vi "solar_voy Get Bits (COSMOS).vi"(6 "Bit Element Size (Array only)":i32, 7 "Endian (BIG)":enum8{"BIG", "LITTLE"}(ring), 8 "COSMOS TYPE":T1, 9 "Bit Size":i32, 10 "Bit Offset":i32, 11 "COSMOS Data":string) -> (2 "Bit Offset Past Value":i32, 3 "LabVIEW Flattened Value":string)   [LabVIEW 2018]
doc: "This unpacks the COSMOS Data given the bit offset and bit size into a LabVIEW Flattened Value."
uses:
  solar_voy_def/solar_voy_def_ctl ITEM TYPE.ctl
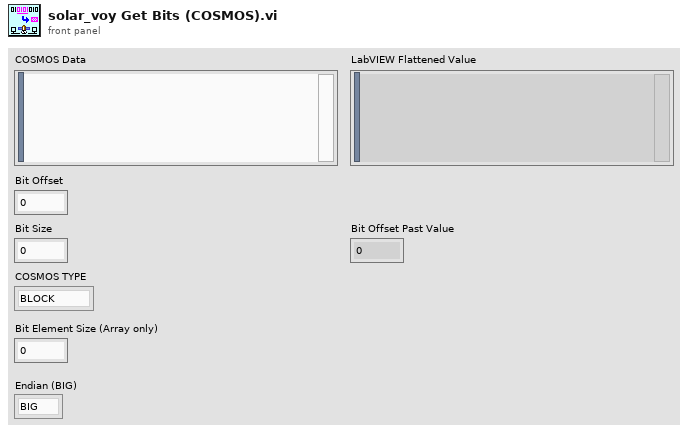
[diagram p1: front panel]
types:
  T1 = typedef "solar_voy_def_ctl ITEM TYPE.ctl" = enum8{"BLOCK", "INT", "UINT", "FLOAT", "STRING"}
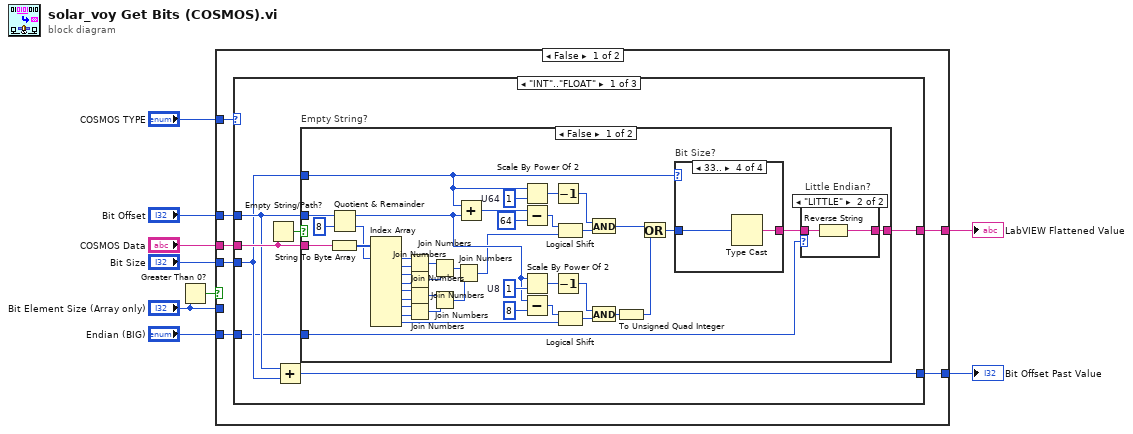
[diagram p0: block diagram]
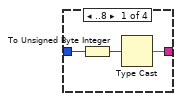
[diagram p3: hidden frame]
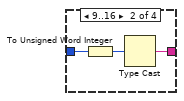
[diagram p4: hidden frame]
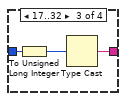
[diagram p5: hidden frame]
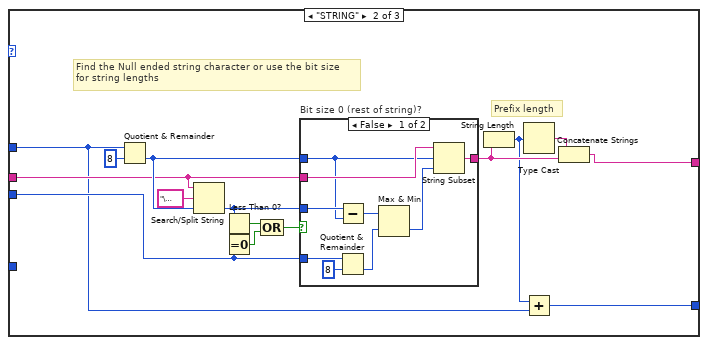
[diagram p7: hidden frame]
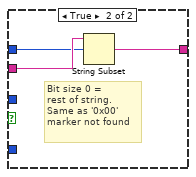
[diagram p8: hidden frame]
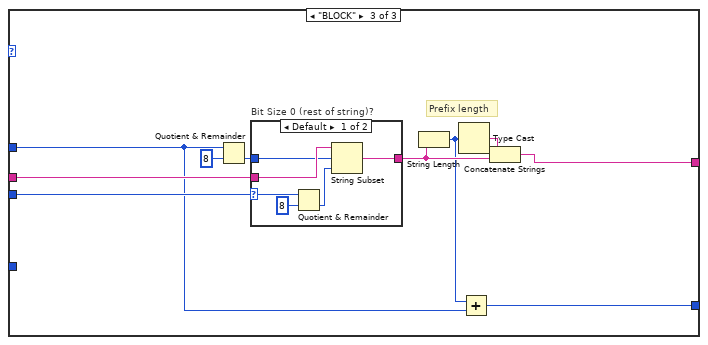
[diagram p9: hidden frame]
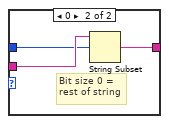
[diagram p10: hidden frame]
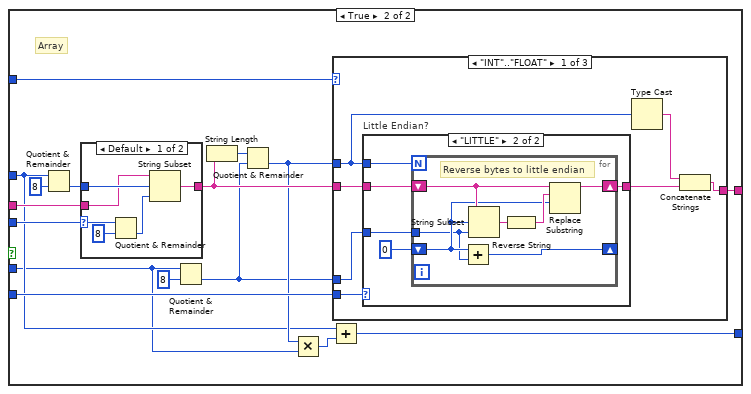
[diagram p11: hidden frame]
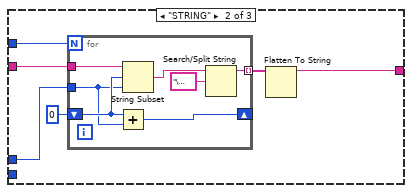
[diagram p13: hidden frame]
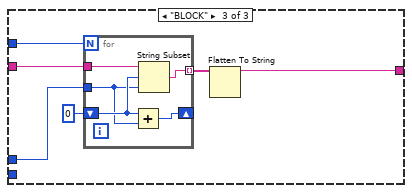
[diagram p14: hidden frame]
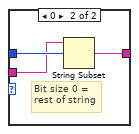
[diagram p15: hidden frame]
diagram:
  n1 = Greater Than 0?(x="Bit Element Size (Array only)") -> (x > 0?=w1:bool)
  n2 = case shown="False" w1 {
    tunnel: "COSMOS Data" -> [w16 w140]
    tunnel: [w15 w136] -> w8
    tunnel: "Bit Offset" -> [w14 w129]
    tunnel: "Bit Size" -> [w13 w139]
    tunnel: [w12 w128] -> w5
    tunnel: "COSMOS TYPE" -> [w11 w137]
    tunnel: "Endian (BIG)" -> [w10 w135]
    tunnel: "Bit Element Size (Array only)" -> [_ w127]
    frame False {
      n3 = case shown="\"INT\"..\"FLOAT\"" w11 {
        tunnel: w16 -> [w23 w88 w115]
        tunnel: [w22 w85 w111] -> w15
        tunnel: w14 -> [w21 w82 w109]
        tunnel: w13 -> [w20 w87 w112]
        tunnel: [w19 w81 w108] -> w12
        tunnel: w10 -> [w17 _ _]
        frame "INT".."FLOAT" {
          n4 = Empty String/Path?(string/path=w23) -> (empty?=w18:bool)
          n5 = Add(x=w21, y=w20) -> (x+y=w19:i32)
          n6 = case "Empty String?" shown="False" w18 {
            tunnel: w23 -> [w55 _]
            tunnel: [w25 _] -> w22
            tunnel: w21 -> [w65 _]
            tunnel: w20 -> [w64 _]
            tunnel: w17 -> [w24 _]
            frame False {
              w38 = u8 1  # U8
              w59 = u64 1  # U64
              n7 = String To Byte Array(string=w55) -> (unsigned byte array=w54:u8[])
              n8 = Quotient & Remainder(x=w65, y=8) -> (x-y*floor(x/y)=w37:i32, floor(x/y)=w27:i32)
              n9 = Index Array(array=w54, index #1=w27) -> (element #1=w53:u8, element #2=w52:u8, element #3=w51:u8, element #4=w50:u8, element #5=w49:u8, element #6=w48:u8, element #7=w47:u8, element #8=w46:u8, element #9=w33:u8)  [unwired: 8 in]
              n10 = Join Numbers(hi=w53, lo=w52) -> ((hi.lo)=w45:u16)
              n11 = Join Numbers(hi=w51, lo=w50) -> ((hi.lo)=w43:u16)
              n12 = Join Numbers(hi=w49, lo=w48) -> ((hi.lo)=w44:u16)
              n13 = Join Numbers(hi=w47, lo=w46) -> ((hi.lo)=w42:u16)
              n14 = Join Numbers(hi=w45, lo=w43) -> ((hi.lo)=w41:u32)
              n15 = Join Numbers(hi=w44, lo=w42) -> ((hi.lo)=w40:u32)
              n16 = Join Numbers(hi=w41, lo=w40) -> ((hi.lo)=w26:u64)
              n17 = Add(x=w64, y=w37) -> (x+y=w62:i32)
              n18 = Scale By Power Of 2(n=w64, x=w59) -> (x*2^n=w58:u64)
              n19 = Subtract(x=w62, y=64) -> (x-y=w56:i32)
              n20 = Scale By Power Of 2(n=w37, x=w38) -> (x*2^n=w39:u8)
              n21 = Subtract(x=w37, y=8) -> (x-y=w34:i32)
              n22 = Decrement(x=w58) -> (x-1=w57:u64)
              n23 = Decrement(x=w39) -> (x-1=w35:u8)
              n24 = Logical Shift(y=w56, x=w26) -> (x << y=w60:u64)
              n25 = Logical Shift(y=w34, x=w33) -> (x << y=w32:u8)
              n26 = And(x=w57, y=w60) -> (x .and. y?=w29:u64)
              n27 = And(x=w35, y=w32) -> (x .and. y?=w31:u8)
              n28 = To Unsigned Quad Integer(1:w31) -> (0:w30:u64)
              n29 = Or(x=w29, y=w30) -> (x .or. y?=w28:u64)
              n30 = case "Bit Size?" shown="33.." w64 {
                tunnel: [w72 w75 w78 w80] -> w66
                tunnel: w28 -> [w71 w74 w77 w79]
                frame ..8 {
                  n31 = To Unsigned Byte Integer(number=w71) -> (unsigned 8bit integer=w70:u8)
                  n32 = Type Cast(x=w70) -> (*(type *) &x=w72:string)  [unwired: 1 in]
                }
                frame 9..16 {
                  n33 = To Unsigned Word Integer(number=w74) -> (unsigned 16bit integer=w73:u16)
                  n34 = Type Cast(x=w73) -> (*(type *) &x=w75:string)  [unwired: 1 in]
                }
                frame 17..32 {
                  n35 = To Unsigned Long Integer(number=w77) -> (unsigned 32bit integer=w76:u32)
                  n36 = Type Cast(x=w76) -> (*(type *) &x=w78:string)  [unwired: 1 in]
                }
                frame 33.. {
                  n37 = Type Cast(x=w79) -> (*(type *) &x=w80:string)  [unwired: 1 in]
                }
              }
              n38 = case "Little Endian?" shown="\"LITTLE\"" w24 {
                tunnel: w66 -> [w67 w69]
                tunnel: [w67 w68] -> w25
                frame "BIG", Default {
                }
                frame "LITTLE" {
                  n39 = Reverse String(1:w69) -> (0:w68:string)
                }
              }
            }
            frame True {
            }
          }
        }
        frame "STRING" {
          # "Find the Null ended string character or use the bit size\nfor string lengths"
          # "Prefix length"
          n40 = Quotient & Remainder(x=w82, y=8) -> (floor(x/y)=w93:i32)  [unwired: 1 out]
          n41 = Search/Split String(string=w88, search string/char (-)="\u0000", offset (0)=w93) -> (offset of match=w92:i32)  [unwired: 2 out]
          n42 = Less Than 0?(x=w92) -> (x < 0?=w91:bool)
          n43 = Equal To 0?(x=w87) -> (x = 0?=w90:bool)
          n44 = Compound Arithmetic op=OR(w91, w90) -> (w89:bool)
          n45 = case "Bit size 0 (rest of string)?" shown="False" w89 {
            tunnel: w88 -> [w104 w107]
            tunnel: w92 -> [w103 _]
            tunnel: w93 -> [w102 w106]
            tunnel: [w97 w105] -> w84
            tunnel: w87 -> [w96 _]
            frame False {
              n46 = Subtract(x=w103, y=w102) -> (x-y=w100:i32)
              n47 = Quotient & Remainder(x=w96, y=8) -> (floor(x/y)=w99:i32)  [unwired: 1 out]
              n48 = Max & Min(x=w100, y=w99) -> (min(x,y)=w98:i32)  [unwired: 1 out]
              n49 = String Subset(string=w104, offset (0)=w102, length (rest)=w98) -> (substring=w97:string)
            }
            frame True {
              # "Bit size 0 =\nrest of string.\nSame as '0x00'\nmarker not found"
              n50 = String Subset(string=w107, offset (0)=w106) -> (substring=w105:string)  [unwired: 1 in]
            }
          }
          n51 = String Length(string=w84) -> (length=w83:i32)
          n52 = Type Cast(x=w83) -> (*(type *) &x=w86:string)  [unwired: 1 in]
          n53 = Add(x=w83, y=w82) -> (x+y=w81:i32)
          n54 = Concatenate Strings(w86, w84) -> (w85:string)
        }
        frame "BLOCK" {
          # "Prefix length"
          n55 = Quotient & Remainder(x=w109, y=8) -> (floor(x/y)=w116:i32)  [unwired: 1 out]
          n56 = case "Bit Size 0 (rest of string)?" shown="Default" w112 {
            selector: w112 -> [w118 _]
            tunnel: w115 -> [w123 w126]
            tunnel: w116 -> [w122 w124]
            tunnel: [w121 w125] -> w113
            frame Default {
              n57 = Quotient & Remainder(x=w118, y=8) -> (floor(x/y)=w120:i32)  [unwired: 1 out]
              n58 = String Subset(string=w123, offset (0)=w122, length (rest)=w120) -> (substring=w121:string)
            }
            frame 0 {
              # "Bit size 0 =\nrest of string"
              n59 = String Subset(string=w126, offset (0)=w124) -> (substring=w125:string)  [unwired: 1 in]
            }
          }
          n60 = String Length(string=w113) -> (length=w110:i32)
          n61 = Type Cast(x=w110) -> (*(type *) &x=w114:string)  [unwired: 1 in]
          n62 = Add(x=w110, y=w109) -> (x+y=w108:i32)
          n63 = Concatenate Strings(w114, w113) -> (w111:string)
        }
      }
    }
    frame True {
      # "Array"
      n64 = Quotient & Remainder(x=w129, y=8) -> (floor(x/y)=w142:i32)  [unwired: 1 out]
      n65 = case shown="Default" w139 {
        selector: w139 -> [w187 _]
        tunnel: w142 -> [w192 w195]
        tunnel: w140 -> [w190 w194]
        tunnel: [w189 w193] -> w133
        frame Default {
          n66 = Quotient & Remainder(x=w187, y=8) -> (floor(x/y)=w188:i32)  [unwired: 1 out]
          n67 = String Subset(string=w190, offset (0)=w192, length (rest)=w188) -> (substring=w189:string)
        }
        frame 0 {
          # "Bit size 0 =\nrest of string"
          n68 = String Subset(string=w194, offset (0)=w195) -> (substring=w193:string)  [unwired: 1 in]
        }
      }
      n69 = Quotient & Remainder(x=w127, y=8) -> (floor(x/y)=w131:i32)  [unwired: 1 out]
      n70 = String Length(string=w133) -> (length=w134:i32)
      n71 = Quotient & Remainder(x=w134, y=w131) -> (floor(x/y)=w132:i32)  [unwired: 1 out]
      n72 = Multiply(x=w132, y=w127) -> (x*y=w130:i32)
      n73 = Add(x=w129, y=w130) -> (x+y=w128:i32)
      n74 = case shown="\"INT\"..\"FLOAT\"" w137 {
        tunnel: [w148 w166 w179] -> w136
        tunnel: w131 -> [w145 w168 w181]
        tunnel: w133 -> [w144 w165 w178]
        tunnel: w135 -> [w146 _ _]
        tunnel: w132 -> [w143 w163 w176]
        frame "INT".."FLOAT" {
          n75 = case "Little Endian?" shown="\"LITTLE\"" w146 {
            tunnel: w144 -> [w150 w154]
            tunnel: [w150 w153] -> w147
            tunnel: w145 -> [_ w152]
            tunnel: w143 -> [_ w151]
            frame "BIG", Default {
            }
            frame "LITTLE" {
              n76 = for {
                N: w151 -> [_]
                shift-right: [w159] -> w153
                shift-left: w154 -> [w160]
                shift-right: [w162] -> _
                shift-left: 0 -> [w157]
                tunnel: w152 -> [w156]
                # "Reverse bytes to little endian"
                n77 = Add(x=w157, y=w156) -> (x+y=w162:i32)
                n78 = String Subset(string=w160, offset (0)=w157, length (rest)=w156) -> (substring=w161:string)
                n79 = Reverse String(1:w161) -> (0:w158:string)
                n80 = Replace Substring(3:w157, 4:w158, 5:w160) -> (1:w159:string)  [unwired: 1 in, 1 out]
              }
            }
          }
          n81 = Type Cast(x=w143) -> (*(type *) &x=w149:string)  [unwired: 1 in]
          n82 = Concatenate Strings(w149, w147) -> (w148:string)
        }
        frame "STRING" {
          n83 = for {
            N: w163 -> [_]
            tunnel: w168 -> [w172]
            tunnel: w165 -> [w175]
            shift-right: [w173] -> _
            shift-left: 0 -> [w174]
            tunnel: [w169] -> w167 mode=indexing
            n84 = Add(x=w174, y=w172) -> (x+y=w173:i32)
            n85 = String Subset(string=w175, offset (0)=w174, length (rest)=w172) -> (substring=w170:string)
            n86 = Search/Split String(string=w170, search string/char (-)="\u0000") -> (substring before match=w169:string)  [unwired: 3 out]
          }
          n87 = Flatten To String(anything=w167) -> (data string=w166:string)  [unwired: 3 in, 2 out]
        }
        frame "BLOCK" {
          n88 = for {
            N: w176 -> [_]
            tunnel: w181 -> [w183]
            tunnel: w178 -> [w186]
            shift-right: [w184] -> _
            shift-left: 0 -> [w185]
            tunnel: [w182] -> w180 mode=indexing
            n89 = Add(x=w185, y=w183) -> (x+y=w184:i32)
            n90 = String Subset(string=w186, offset (0)=w185, length (rest)=w183) -> (substring=w182:string)
          }
          n91 = Flatten To String(anything=w180) -> (data string=w179:string)  [unwired: 3 in, 2 out]
        }
      }
    }
  }
  "LabVIEW Flattened Value" <- w8
  "Bit Offset Past Value" <- w5
